vi "Add Admin Passwordv2.vi"(8 "error in (no error)":errorcluster, 10 "Write Password":string, 11 "Masterv2 in":refnum<class "Masterv2.lvclass">) -> (0 "error out":errorcluster, 3 "Masterv2 out":refnum<class "Masterv2.lvclass">)   [LabVIEW 2014, in "Main Libraryv2.lvlib" / "Masterv2.lvclass"]
uses:
  Master/Masterv2.lvclass
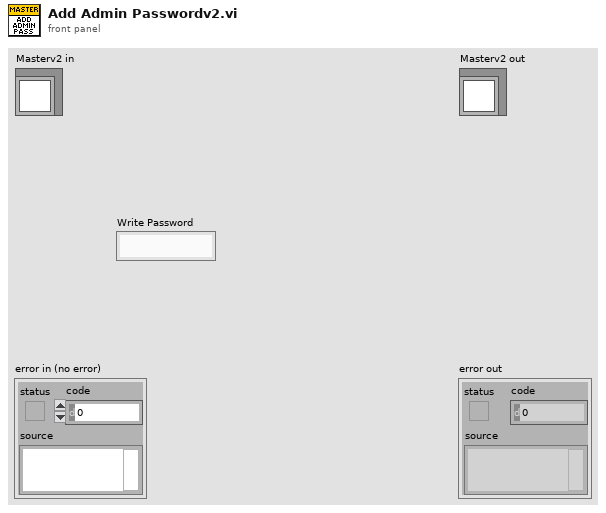
[diagram p1: front panel]
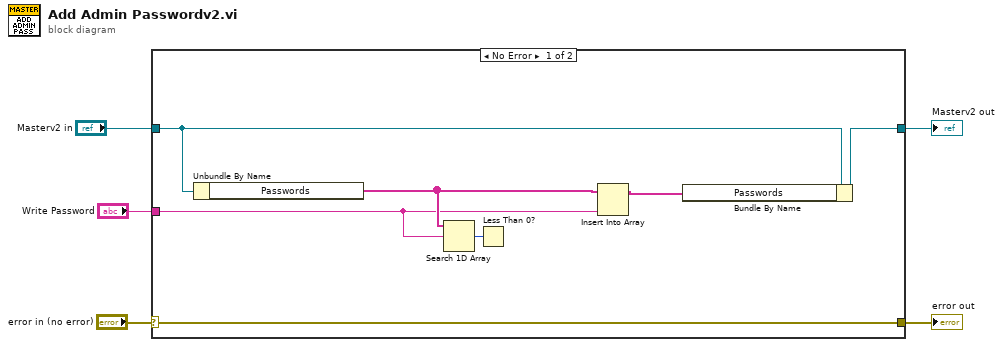
[diagram p0: block diagram]
diagram:
  n1 = case shown="No Error" "error in (no error)" {
    selector: "error in (no error)" -> [w12 w14]
    tunnel: [w12 w14] -> w4
    tunnel: [w6 w13] -> w2
    tunnel: "Masterv2 in" -> [w7 w13]
    tunnel: "Write Password" -> [w8 _]
    frame No Error {
      n2 = Unbundle By Name(w7) -> ("Passwords"=w10:string[])
      n3 = Search 1D Array(1D array=w10, element=w8) -> (index of element=w11:i32)  [unwired: 1 in]
      n4 = Less Than 0?(x=w11) -> ()  [unwired: 1 out]
      n5 = Insert Into Array(array=w10, new element=w8) -> (w9:string[])  [unwired: 1 in]
      n6 = Bundle By Name(cluster=w7, "Passwords"=w9) -> (w6:refnum<class "Masterv2.lvclass">)
    }
    frame Error {
    }
  }
  "error out" <- w4
  "Masterv2 out" <- w2
